vi "archivo de pruebas.vi"() -> ()   [LabVIEW 2013]
panel:
  out "x + iy":csg
  in  "Numeric":csg
  out "nearest integer value":dbl
  out "Array 2":dbl[](array[numeric])
  out "size(s)":i32
  out "Array":dbl[](array[numeric])
  out "x-y":dbl[](array[numeric])
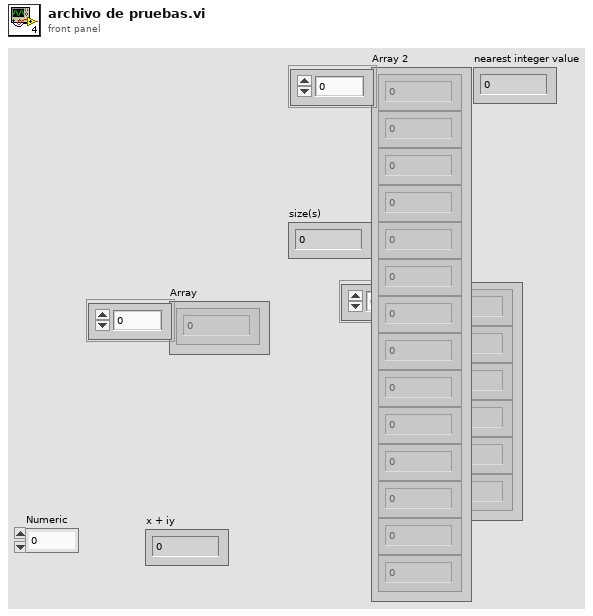
[diagram p1: front panel]
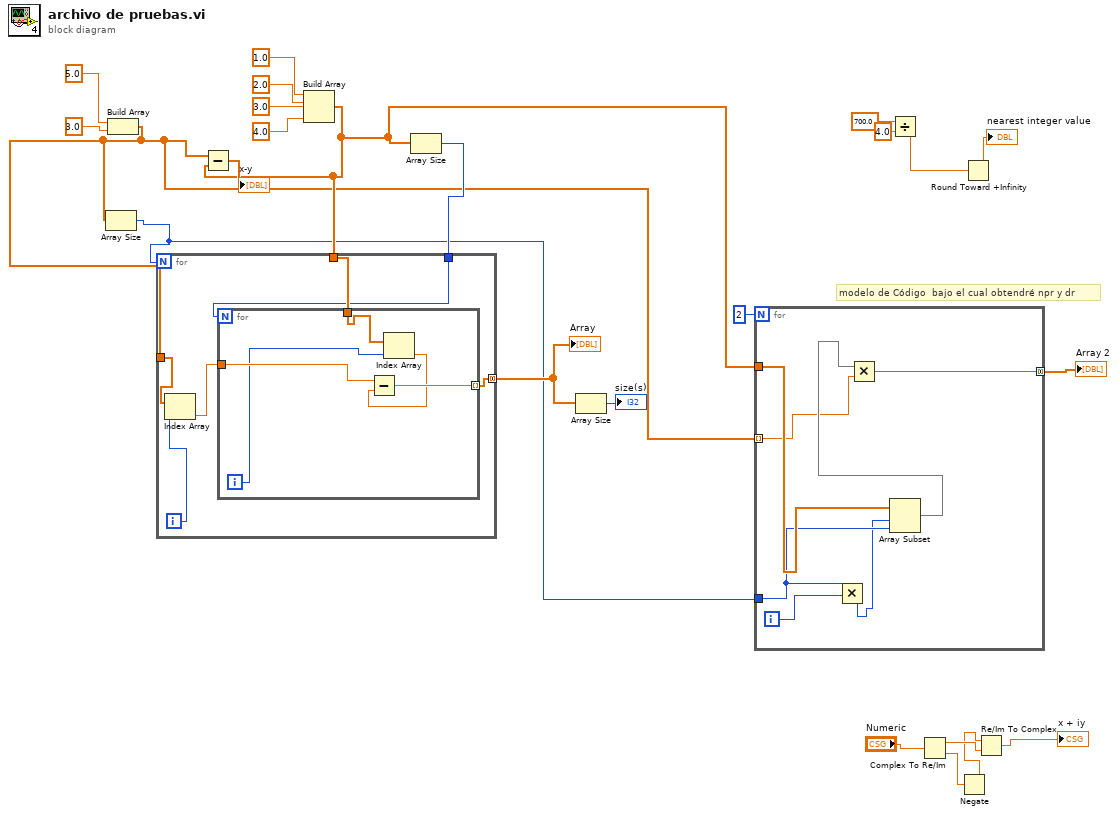
[diagram p0: block diagram]
diagram:
  # "modelo de Código  bajo el cual obtendré npr y dr"
  n1 = Build Array(5.0 ("element"), 3.0 ("element")) -> (w13:dbl[])
  n2 = Array Size(array=w13) -> (size(s)=w10:i32)
  n3 = Build Array(1.0 ("element"), 2.0 ("element"), 3.0 ("element"), 4.0 ("element")) -> (w14:dbl[])
  n4 = Subtract(x=w13, y=w14) -> (x-y=→"x-y":dbl[])
  n5 = Array Size(array=w14) -> (size(s)=w15:i32)
  n6 = for {
    N: w10 -> [_]
    tunnel: w13 -> [w28]
    tunnel: w14 -> [w29]
    tunnel: [w30] -> w17 mode=concatenating
    tunnel: w15 -> [w25]
    i -> [w27]
    n7 = Index Array(array=w28, index=w27) -> (element=w26:dbl)
    n8 = for {
      N: w25 -> [_]
      tunnel: w26 -> [w35]
      tunnel: [w34] -> w30 mode=indexing
      tunnel: w29 -> [w33]
      i -> [w32]
      n9 = Index Array(array=w33, index=w32) -> (element=w31:dbl)
      n10 = Subtract(x=w35, y=w31) -> (x-y=w34:dbl)
    }
  }
  "Array" <- w17
  n11 = Array Size(array=w17) -> (size(s)=→"size(s)":i32)
  n12 = for {
    N: 2 -> [_]
    tunnel: w14 -> [w41]
    tunnel: [w42] -> w12 mode=concatenating
    tunnel: w13 -> [w36] mode=indexing
    tunnel: w10 -> [w38]
    i -> [w39]
    n13 = Multiply(x=w39, y=w38) -> (x*y=w37:i32)
    n14 = Array Subset(array=w41, index=w37, length=w38) -> (w40:dbl[])
    n15 = Multiply(x=w40, y=w36) -> (x*y=w42:dbl[])
  }
  "Array 2" <- w12
  n16 = Divide(x=700.0, y=4.0) -> (x/y=w7:dbl)
  n17 = Complex To Re/Im(x + iy="Numeric") -> (x=w2:sgl, y=w3:sgl)
  n18 = Negate(x=w3) -> (-x=w1:sgl)
  n19 = Round Toward +Infinity(x=w7) -> (ceil(x): smallest int >= x=→"nearest integer value":dbl)
  n20 = Re/Im To Complex(1:w2, 2:w1) -> (0:→"x + iy":csg)
